vi "main.vi"() -> ()   [LabVIEW 2016]
doc: "Model Isinga 2D\nSebastian Rochacki nr indeksu (236 617)"
uses:
  <vilib>/Analysis/Matrix/Datatypes/RealMatrix.ctl
  <vilib>/express/express arith-compare/Formula/XNode/ExpressFormulaBlockNode.xnode
  <vilib>/Analysis/Matrix/NI_Matrix.lvlib
panel:
  in  "Tab Control":enum32{"Konfiguracje", "Magnetyzacja"}(tab)
  out "Konfiguracje symulowanego układu, wartości węzłów s(i,j) = + - 1":dbl[][](graph)
  out "Zależność magnetyzacji od liczby kroków Monte Carlo":cluster{"Y":dbl[], "Y":dbl[]}[](graph)
  in  "?":bool
  out "Magnetyzacja suma":dbl
  out "Magnetyzacja średnia symulowanego\nukładu (miara uporządkowania)":dbl format="%#.2g"
  out "licznik":i32
  in  "Symulacja":bool
  in  "stop":bool
  in  "Wielkość siatki":i32=10 min=5 max=100 step=5
  in  "Temperatura zredukowana":dbl=1.5 min=1.0 max=5.0 step=0.1 format="%#_2g"
  in  "Macierz węzłów":T1
  # "Model Isinga 2D"
  # "Parametry początkowe:"
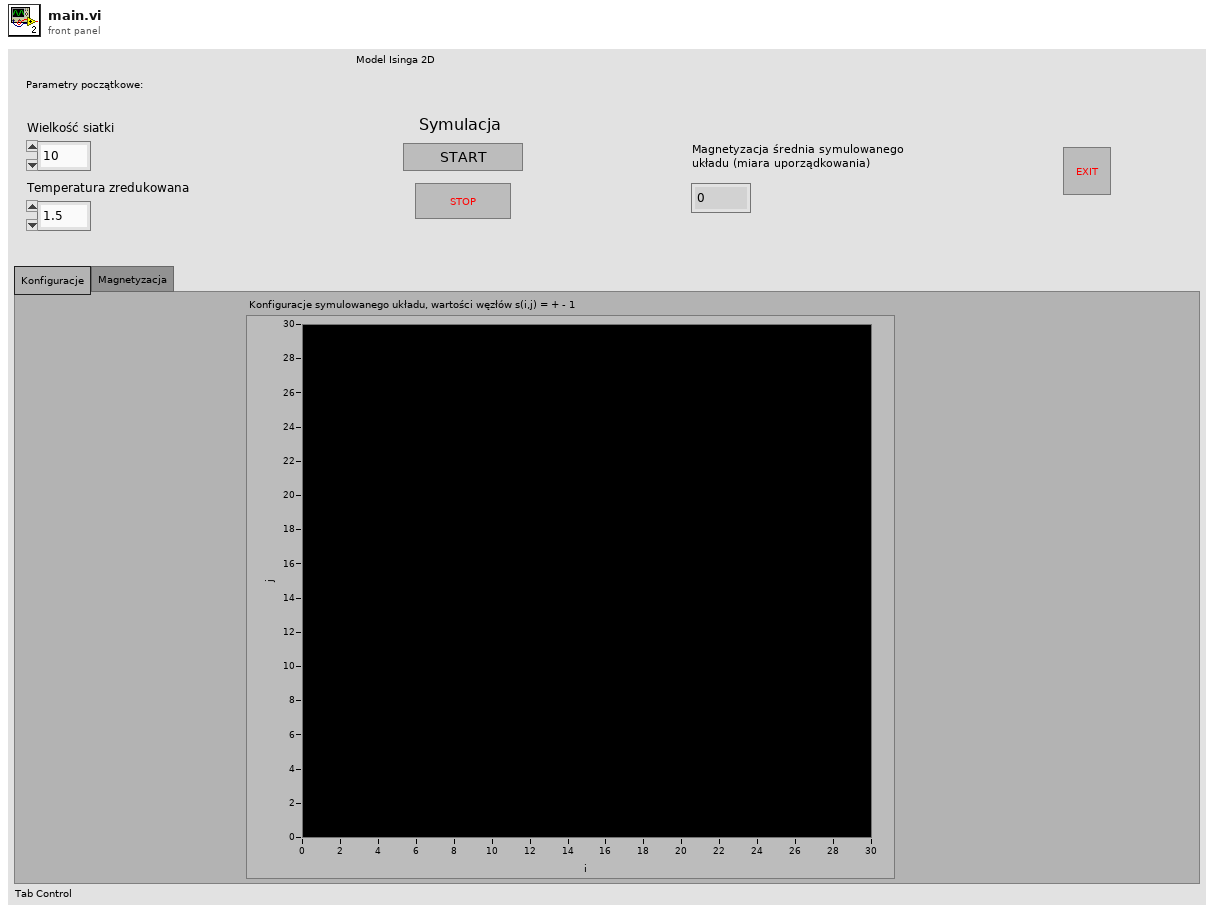
[diagram p1: front panel]
types:
  T1 = typedef "NI_Matrix.lvlib/RealMatrix.ctl" = dbl[][]
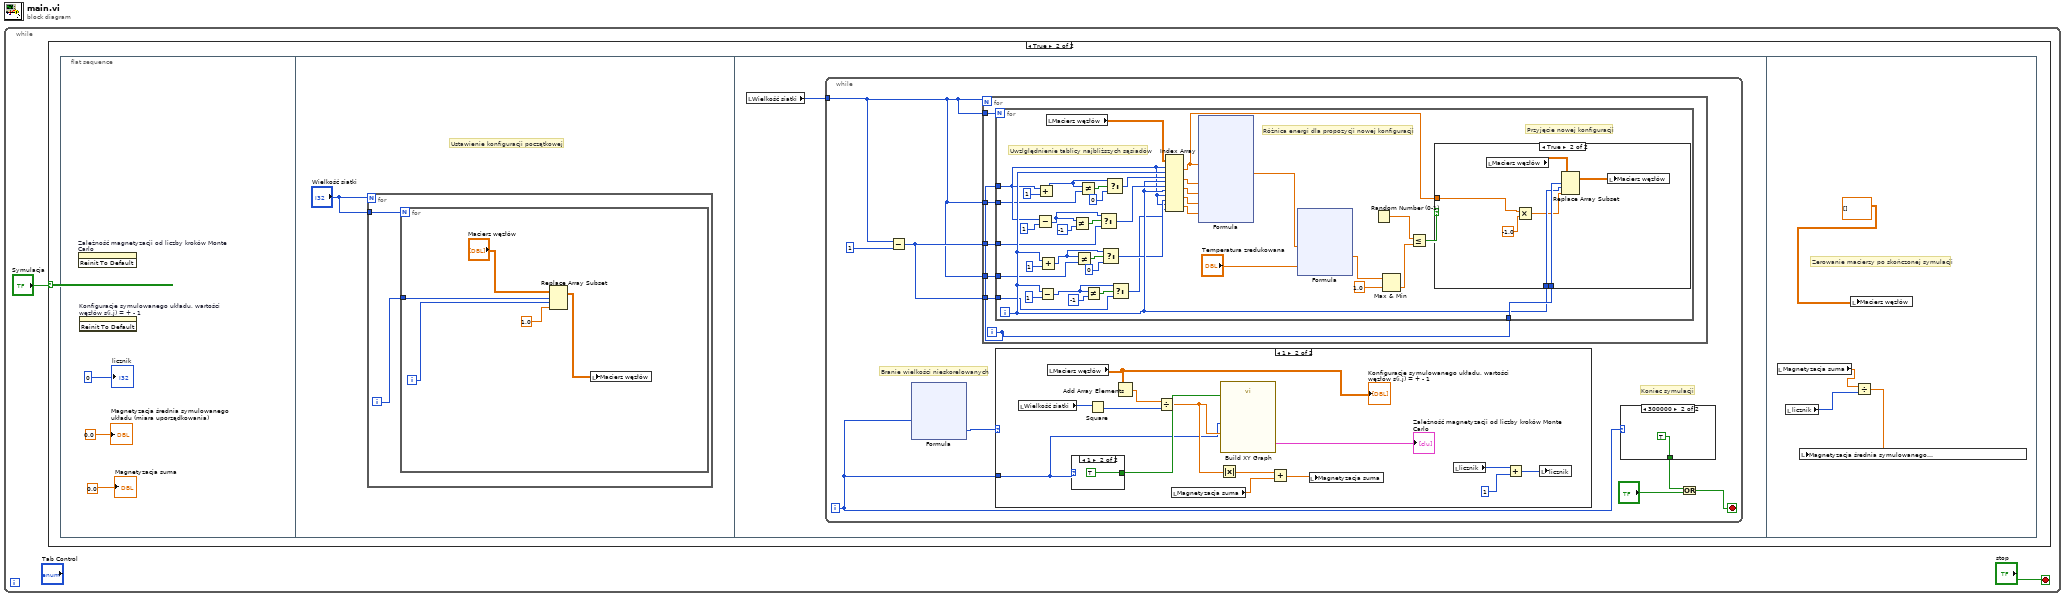
[diagram p0: block diagram]
diagram:
  n1 = while {
    stop <- "stop" stop-if-true
    n2 = case shown="True" "Symulacja" {
      frame False {
      }
      frame True {
        n3 = flat-sequence {
          frame #0 {
            n4 = invoke on="Zależność magnetyzacji od liczby kroków Monte Carlo" class="XYGraph (strict)" method="Reinit To Default"() -> ()  [unwired: 3 in, 3 out]
            n5 = invoke on="Konfiguracje symulowanego układu, wartości węzłów s(i,j) = + - 1" class="IntGraph (strict)" method="Reinit To Default"() -> ()  [unwired: 3 in, 3 out]
            "licznik" <- 0 ("licznik")
            "Magnetyzacja średnia symulowanego\nukładu (miara uporządkowania)" <- 0.0 ("<m>")
            "Magnetyzacja suma" <- 0.0 ("Magnetyzacja suma")
          }
          frame #1 {
            # "Ustawienie konfiguracji początkowej"
            n6 = for {
              N: "Wielkość siatki" -> [_]
              tunnel: "Wielkość siatki" -> [w7]
              i -> [w8]
              n7 = for {
                N: w7 -> [_]
                tunnel: w8 -> [w13]
                i -> [w9]
                n8 = Replace Array Subset(array="Macierz węzłów", new element=1.0 ("new element/submatrix"), index (row)=w13, index (col)=w9) -> (w10:T1)
                n9 = local write "Macierz węzłów"(w10) -> ()
              }
            }
          }
          frame #2 {
            n10 = local read "Wielkość siatki"() -> (w14:i32)
            n11 = while {
              tunnel: w14 -> [w19]
              i -> [w18]
              stop <- w15 stop-if-true
              # "Koniec symulacji"
              # "Branie wielkości nieskorelowanych"
              n12 = Subtract(x=w19, y=1) -> (x-y=w20:i32)
              n13 = xnode "Formula"("X1"=w18) -> ("Result"=w22:i32)  [unwired: 1 in, 1 out]
              n14 = for {
                N: w19 -> [_]
                tunnel: w20 -> [w51]
                tunnel: w20 -> [w50]
                tunnel: w19 -> [w49]
                tunnel: w19 -> [w48]
                tunnel: w19 -> [w47]
                i -> [w52]
                n15 = for {
                  N: w49 -> [_]
                  tunnel: w52 -> [w86]
                  tunnel: w52 -> [w67]
                  tunnel: w51 -> [w56]
                  tunnel: w50 -> [w55]
                  tunnel: w48 -> [w54]
                  tunnel: w47 -> [w53]
                  i -> [w72]
                  # "Różnica energi dla propozycji nowej konfiguracji"
                  # "Uwzlględnienie tablicy najbliższych sąsiadów"
                  # "Przyjęcie nowej konfiguracji"
                  n16 = Subtract(x=w67, y=1) -> (x-y=w74:i32)
                  n17 = Add(x=w67, y=1) -> (x+y=w78:i32)
                  n18 = Subtract(x=w72, y=1) -> (x-y=w64:i32)
                  n19 = Add(x=w72, y=1) -> (x+y=w69:i32)
                  n20 = local read "Macierz węzłów"() -> (w57:T1)
                  n21 = Not Equal?(x=w74, y=-1) -> (x != y?=w76:bool)
                  n22 = Not Equal?(x=w69, y=w53) -> (x != y?=w70:bool)
                  n23 = Not Equal?(x=w78, y=w54) -> (x != y?=w79:bool)
                  n24 = Not Equal?(x=w64, y=-1) -> (x != y?=w66:bool)
                  n25 = Select(t=w74, s=w76, f=w55) -> (s? t:f=w73:i32)
                  n26 = Select(t=w69, s=w70, f=0) -> (s? t:f=w68:i32)
                  n27 = Select(t=w78, s=w79, f=0) -> (s? t:f=w77:i32)
                  n28 = Select(t=w64, s=w66, f=w56) -> (s? t:f=w63:i32)
                  n29 = Index Array ("Get Matrix Elements")(array=w57, index (row) #1=w67, index (col) #1=w72, index (row) #2=w77, index (col) #2=w72, index (row) #3=w73, index (col) #3=w72, index (row) #4=w67, index (col) #4=w68, index (row) #5=w67, index (col) #5=w63) -> (element #1=w58:dbl, element #2=w62:dbl, element #3=w61:dbl, element #4=w60:dbl, element #5=w59:dbl)
                  n30 = xnode "Formula"("X1"=w58, "X2"=w62, "X3"=w61, "X4"=w60, "X5"=w59) -> ("Result"=w92:dbl)  [unwired: 1 in, 1 out]
                  n31 = xnode "Formula"("X1"=w92, "X2"="Temperatura zredukowana") -> ("Result"=w90:dbl)  [unwired: 1 in, 1 out]
                  n32 = Random Number (0-1)() -> (number: 0 to 1=w88:dbl)
                  n33 = Max & Min(x=w90, y=1.0) -> (min(x,y)=w87:dbl)  [unwired: 1 out]
                  n34 = Less Or Equal?(x=w88, y=w87) -> (x <= y?=w85:bool)
                  n35 = case shown="True" w85 {
                    tunnel: w86 -> [_ w97]
                    tunnel: w72 -> [_ w96]
                    tunnel: w58 -> [_ w93]
                    frame False {
                    }
                    frame True {
                      n36 = local read "Macierz węzłów"() -> (w98:T1)
                      n37 = Multiply ("Multiply.vi")(x=w93, y=-1.0) -> (x*y=w95:dbl)
                      n38 = Replace Array Subset(array=w98, new element=w95, index (row)=w97, index (col)=w96) -> (w99:T1)
                      n39 = local write "Macierz węzłów"(w99) -> ()
                    }
                  }
                }
              }
              n40 = case shown="1" w22 {
                tunnel: w18 -> [_ w32]
                frame 0, Default {
                }
                frame 1 {
                  n41 = local read "Wielkość siatki"() -> (w44:i32)
                  n42 = local read "Macierz węzłów"() -> (w42:T1)
                  "Konfiguracje symulowanego układu, wartości węzłów s(i,j) = + - 1" <- w42
                  n43 = case shown="1" w32 {
                    tunnel: [_ TRUE ("Reset")] -> w40
                    frame 0, Default {
                    }
                    frame 1 {
                    }
                  }
                  n44 = Square(x=w44) -> (x^2=w43:i32)
                  n45 = Add Array Elements(numeric array=w42) -> (sum=w45:dbl)
                  n46 = Divide(x=w45, y=w43) -> (x/y=w38:dbl)
                  n47 = local read "Magnetyzacja suma"() -> (w36:dbl)
                  n48 = Absolute Value(x=w38) -> (abs(x)=w37:dbl)
                  n49 = call "Build XY Graph"("Reset"=w40, "Y Input"=w38, "X Input"=w32) -> ("XY Graph"=→"Zależność magnetyzacji od liczby kroków Monte Carlo":cluster{"X":dbl[], "Y":dbl[]}[])  [unwired: 7 in, 1 out]
                  n50 = Add(x=w37, y=w36) -> (x+y=w35:dbl)
                  n51 = local write "Magnetyzacja suma"(w35) -> ()
                  n52 = local read "licznik"() -> (w34:i32)
                  n53 = Add(x=w34, y=1 ("x")) -> (x+y=w39:i32)
                  n54 = local write "licznik"(w39) -> ()
                }
              }
              n55 = case shown="300000" w18 {
                tunnel: [_ TRUE ("stop 2")] -> w17
                frame 0, Default {
                }
                frame 300000 {
                }
              }
              n56 = Or(x=w17, y="?") -> (x .or. y?=w15:bool)
            }
          }
          frame #3 {
            # "Zerowanie macierzy po skończonej symulacji"
            n57 = local read "Magnetyzacja suma"() -> (w126:dbl)
            n58 = local read "licznik"() -> (w127:i32)
            n59 = local write "Macierz węzłów"(T1 [] ("Macierz przechowująca wartości węzłów = +- 1")) -> ()
            n60 = Divide(x=w126, y=w127) -> (x/y=w128:dbl)
            n61 = local write "Magnetyzacja średnia symulowanego\nukładu (miara uporządkowania)"(w128) -> ()
          }
        }
      }
    }
  }
